vi "SW_Gen_Get_Bounding_rectangles.vi"(3 "Draw Area Size":cluster{"Width":dbl, "Height":dbl}, 4 "Cluster of image geometrical and scaling parameters":T2) -> (1 "Bounding rectangles":T1)   [LabVIEW 2018]
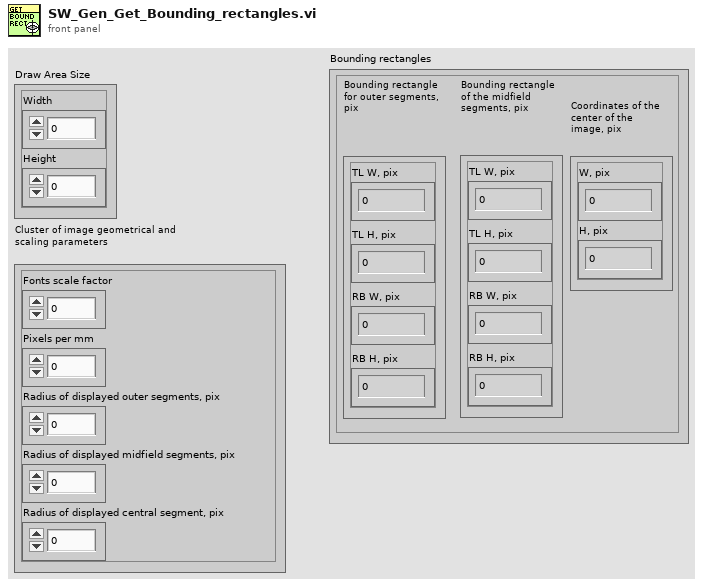
[diagram p1: front panel]
types:
  T1 = cluster{"Bounding rectangle for outer segments, pix":cluster{"TL W, pix":dbl, "TL H, pix":dbl, "RB W, pix":dbl, "RB H, pix":dbl}, "Bounding rectangle of the midfield segments, pix":cluster{"TL W, pix":dbl, "TL H, pix":dbl, "RB W, pix":dbl, "RB H, pix":dbl}, "Coordinates of the center of the image, pix":cluster{"W, pix":dbl, "H, pix":dbl}}
  T2 = cluster{"Fonts scale factor":dbl, "Pixels per mm":dbl, "Radius of displayed outer segments, pix":dbl, "Radius of displayed midfield segments, pix":dbl, "Radius of displayed central segment, pix":dbl}
  T3 = cluster{cluster{dbl, dbl, dbl, dbl}, cluster{dbl, dbl, dbl, dbl}, cluster{dbl, dbl}}
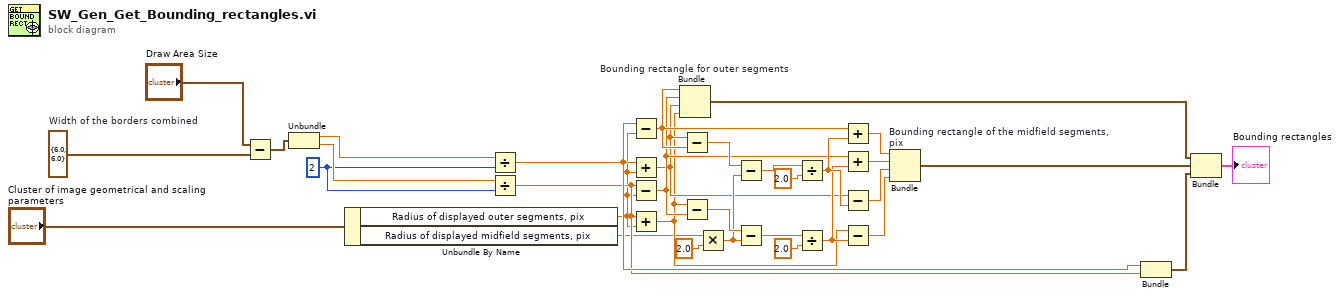
[diagram p0: block diagram]
diagram:
  w29 = cluster{"Width":dbl, "Height":dbl} {"Width"=6.0, "Height"=6.0}  # Width of the borders combined
  w28 = u32 2 ("y")
  n1 = Subtract(x="Draw Area Size", y=w29) -> (x-y=w30:cluster{"Width":dbl, "Height":dbl})
  n2 = Unbundle(w30) -> ("Width"=w32:dbl, "Height"=w33:dbl)
  n3 = Unbundle By Name("Cluster of image geometrical and scaling parameters") -> ("Radius of displayed outer segments, pix"=w2:dbl, "Radius of displayed midfield segments, pix"=w1:dbl)
  n4 = Divide(x=w32, y=w28) -> (x/y=w26:dbl)
  n5 = Divide(x=w33, y=w28) -> (x/y=w25:dbl)
  n6 = Subtract(x=w26, y=w2) -> (x-y=w10:dbl)
  n7 = Add(x=w26, y=w2) -> (x+y=w8:dbl)
  n8 = Subtract(x=w25, y=w2) -> (x-y=w9:dbl)
  n9 = Add(x=w25, y=w2) -> (x+y=w7:dbl)
  n10 = Bundle "Bounding rectangle for outer segments"(w10, w9, w8, w7) -> (w6:cluster{dbl, dbl, dbl, dbl})  [unwired: 1 in]
  n11 = Subtract(x=w8, y=w10) -> (x-y=w24:dbl)
  n12 = Subtract(x=w7, y=w9) -> (x-y=w19:dbl)
  n13 = Multiply(x=w1, y=2.0) -> (x*y=w18:dbl)
  n14 = Subtract(x=w24, y=w18) -> (x-y=w22:dbl)
  n15 = Subtract(x=w19, y=w18) -> (x-y=w16:dbl)
  n16 = Divide(x=w22, y=2.0) -> (x/y=w20:dbl)
  n17 = Divide(x=w16, y=2.0) -> (x/y=w15:dbl)
  n18 = Add(x=w10, y=w20) -> (x+y=w14:dbl)
  n19 = Add(x=w9, y=w15) -> (x+y=w12:dbl)
  n20 = Subtract(x=w8, y=w20) -> (x-y=w13:dbl)
  n21 = Subtract(x=w7, y=w15) -> (x-y=w11:dbl)
  n22 = Bundle "Bounding rectangle of the midfield segments, pix"(w14, w12, w13, w11) -> (w5:cluster{dbl, dbl, dbl, dbl})  [unwired: 1 in]
  n23 = Bundle ("Coordinates of the center of the image")(w26, w25) -> (w4:cluster{dbl, dbl})  [unwired: 1 in]
  n24 = Bundle(w6, w5, w4) -> (→"Bounding rectangles":T3)  [unwired: 1 in]
